vi "Add.vi"(7 "LabVIEW Web Service Request":refnum<class "Web Request.lvclass">, 10 "B":dbl format="%#_13g", 11 "A":dbl format="%#_13g") -> (2 "String":string="Query String", 3 "C":dbl format="%#_13g")   [LabVIEW 2016]
uses:
  <vilib>/wsapi/Web Request.lvclass
panel:
  # "Daniel Smith depaz"
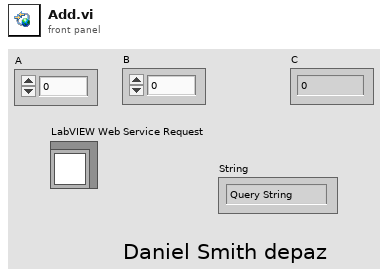
[diagram p1: front panel]
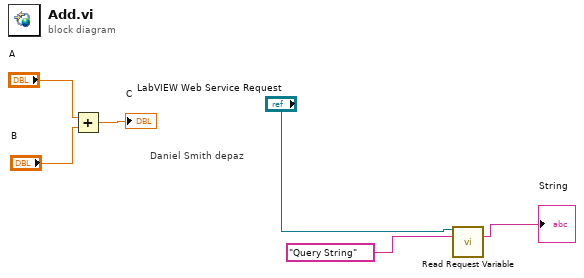
[diagram p0: block diagram]
diagram:
  # "Daniel Smith depaz"
  n1 = Add(x="A", y="B") -> (x+y=→"C":dbl)
  n2 = call <vilib>:"Read Request Variable.vi"("LabVIEW Web Service Request"="LabVIEW Web Service Request", "variable name"="Query String") -> ("value"=→"String":string)  [unwired: 11 in, 2 out]
